vi "Meas_global.vi"() -> ()   [LabVIEW 2010]
uses:
  Controls/Board_Types.ctl
  Controls/Ch_and_Spans.ctl
  Controls/Analysis_info_cluster.ctl
  Controls/Inst_type.ctl
  Controls/Instrument_Array.ctl
  Controls/Graph_Type.ctl
  Controls/Velocity_cluster.ctl
  Controls/Correlation_cluster.ctl
  Controls/Post_Process.ctl
  Controls/Analysis_type_cluster.ctl
  Controls/Analysis_type_Enum.ctl
  Controls/Trigger_Mode.ctl
  Controls/PWA_Data.ctl
panel:
  in  "Iteration Number":i32
  in  "No of Analogue Samples":i32=128 min=0 step=1
  in  "Timescales (s)":dbl[](array[numeric]) format="%.2f"
  in  "Analogue Sampling Rate":dbl
  in  "No of Non Analogue Chs":i32
  in  "PWA Data":T1
  in  "Blocks to Skip":i32[](array[numeric])
  in  "Repeat Measurement?":bool
  in  "Duplicate channels":i32[](array[numeric])
  in  "stop":bool
  out "Flattened data type":enum16{"4.x", "Standard"}(ring)
  in  "Trigger mode":T2
  out "Time Data was Aquired":dbl format="%.2f"
  in  "No of Vari Spaced Chs":i32
  in  "Meas Setup filename":string
  in  "Error Messages":string
  in  "Extra Comments":string
  in  "Requested Sampling rate":dbl=100.0 format="%.2f"
  in  "People to Email":string[](array[string])
  in  "Actual Measurement time (min)":dbl=6.0 format="%.2f"
  in  "Averaging time (min)":dbl=6.0 format="%.2f"
  in  "Continuous time trace?":bool
  in  "Processing last block?":bool
  out "Prog's last revision date":u32
  in  "ADAM Ch Names":string[](array[string])
  in  "LDA frequency":dbl
  in  "Smoothing setups":T3(array[cluster]) {"Y axis"."Format" items=["Decimal", "Scientific", "Engineering"]; "Y axis"."Mapping" items=["Linear", "Logarithmic"]; "X axis"."Format" items=["Decimal", "Scientific", "Engineering"]; "X axis"."Mapping" items=["Linear", "Logarithmic"]}
  in  "Remote control":bool
  out "Analysis type array":T4[](array[typedef])
  out "Current Block No":i32
  in  "New Setup String":string
  in  "Analogue data":enum16{"No Analogue data", "Take Analogue data"}(ring)
  in  "Pre Setup String":string
  in  "interval scanning":bool
  in  "Post Process":T7
  in  "Transit time":bool
  in  "Arrival spacing":bool
  in  "Actual Sampling rate (Hz)":dbl=1000.0 format="%.2f"
  out "Auto-Corr control":i32[](array[numeric])
  out "Spectra control":i32[](array[numeric])
  in  "BSA data rate string":string
  in  "Cross wire + or -ve":T8(ring)
  in  "output polarity":u16(ring)=1 items=["do not change", "positive", "negative"]
  out "Correlation Cluster Array":T9[](array[typedef]) {"u^2w^2" format="%.2f"; "u^3w" format="%.2f"; "uw^3" format="%.2f"; "uw/u'w'" format="%.2f"; "uw^2" format="%.2f"; "u^2w" format="%.2f"; "uw" format="%.2f"}
  out "Velocity Cluster Array":T10[](array[typedef]) {"u^4" format="%.2f"; "Mean % Err" format="%.2f"; "u^4/(u^2)^2 -3" format="%.2f"; "u^3/(u^2)^(1.5)" format="%.2f"; "u^2" format="%.2f"; "% u'/U" format="%.2f"; "U" format="%.2f"}
  in  "LDA data":enum16{"No LDA data", "Take LDA data"}(ring)
  in  "Comments":string
  in  "Over/Under string":string
  in  "Second Graph":T12={"Plot 1"=1, "Plot 2"=3, "Save graph"=0, "Plot Type"=enum."Voltage trace"} {"Save graph" items=["Do not save plot", "Save plot"]; "Plot 2" items=["Nothing", "Velocity1", "Arr time1", "Velocity2", "Arr time2"]; "Plot 1" items=["Nothing", "Velocity1", "Arr time1", "Velocity2", "Arr time2"]}
  in  "First Graph":T12={"Plot 1"=1, "Plot 2"=3, "Save graph"=0, "Plot Type"=enum."Voltage trace"} {"Save graph" items=["Do not save plot", "Save plot"]; "Plot 2" items=["Nothing", "Velocity1", "Arr time1", "Velocity2", "Arr time2"]; "Plot 1" items=["Nothing", "Velocity1", "Arr time1", "Velocity2", "Arr time2"]}
  in  "hist extremes":dbl[][](array[numeric]) format="%.2f"
  out "Histogram control":i32[](array[numeric])
  in  "Bins":i32
  in  "Synchronise with LDA":bool
  in  "No of LDA data channels":i32
  in  "Data Validity":dbl=3.0 min=1.0 max=10.0 format="%.2f"
  out "Diagnostic info":string[][](table)
  in  "correlate":i32[][](array[numeric]) min=0 max=8
  in  "dimensions":enum16{"1D", "2D"}(ring)=enum."2D"
  in  "Raw data file":path
  in  "Analysis Info cluster":T13[](array[typedef])=[{"Colour"=0, "Inst type"=enum."Pitot-static tube", "Inst name"="Manometer voltage", "Symbol"="U", "Code name"="", "Extra Info"="U", "Inst Array"=enum."PWA", "Index"=0, "Voltage Index"=0, "Extra Titles"=[], "Extra Values"=[]}, {"Colour"=0, "Inst type"=enum."Pitot-static tube", "Inst name"="Manometer voltage", "Symbol"="U", "Code name"="", "Extra Info"="U", "Inst Array"=enum."PWA", "Index"=0, "Voltage Index"=0, "Extra Titles"=[], "Extra Values"=[]}, {"Colour"=0, "Inst type"=enum."Pitot-static tube", "Inst name"="Manometer voltage", "Symbol"="U", "Code name"="", "Extra Info"="U", "Inst Array"=enum."PWA", "Index"=0, "Voltage Index"=0, "Extra Titles"=[], "Extra Values"=[]}, {"Colour"=0, "Inst type"=enum."Pitot-static tube", "Inst name"="Manometer voltage", "Symbol"="U", "Code name"="", "Extra Info"="U", "Inst Array"=enum."PWA", "Index"=0, "Voltage Index"=0, "Extra Titles"=[], "Extra Values"=[]}]
  out "Ch & spans + mod limits":T15[](array[typedef]) {"low limit (-10V)" format="%.3f"; "high limit (10V)" format="%.3f"}
  out "Vel stat display":string[][](table)
  in  "Position":T16(array[cluster]) {"Z" format="%.1f"; "Y" format="%.1f"; "X" format="%.1f"}
  in  "Insts for plotting":u16[][](array[ring]) items=["Nothing", "Ref Prop 1", "XW1 1", "XW2 1"]
  in  "Requested No of blocks":i32
  in  "Temp":dbl=20.0 format="%.1f"
  in  "File":T17(ring)
  in  "Results file":path
  in  "Requested No of samples":i32=128 min=0 step=1
  out "Raw data option":enum16{"Save raw data", "Raw data not saved"}(ring)
  out "Start of I16 data (bytes)":i32
  in  "Start Time of experiment":dbl format="%.2f"
  out "Ch & spans":T15[](array[typedef]) {"low limit (-10V)" format="%.3f"; "high limit (10V)" format="%.3f"}
  out "Vel stats info for files":string[](array[string])
  out "Calib file strings":string[](array[string])
  out "Calib consts":dbl[][](array[numeric]) format="%.6f"
  out "Calib type name":string[](array[string])
  out "Calib files":path[](array[path])
  out "Board type":T18=enum."NB-MIO-16H"
  out "Offset voltages":dbl[](array[numeric]) format="%.2f"
  out "Abs Press (mbar)":dbl=1005.0 format="%.2f"
  out "ch info array":dbl[][](array[numeric]) format="%.2f"
  # "LDA information"
  # "File Information"
  # "Analogue input information"
  # "General controls"
  # "Analysis output information"
  # "Analysis setup information"
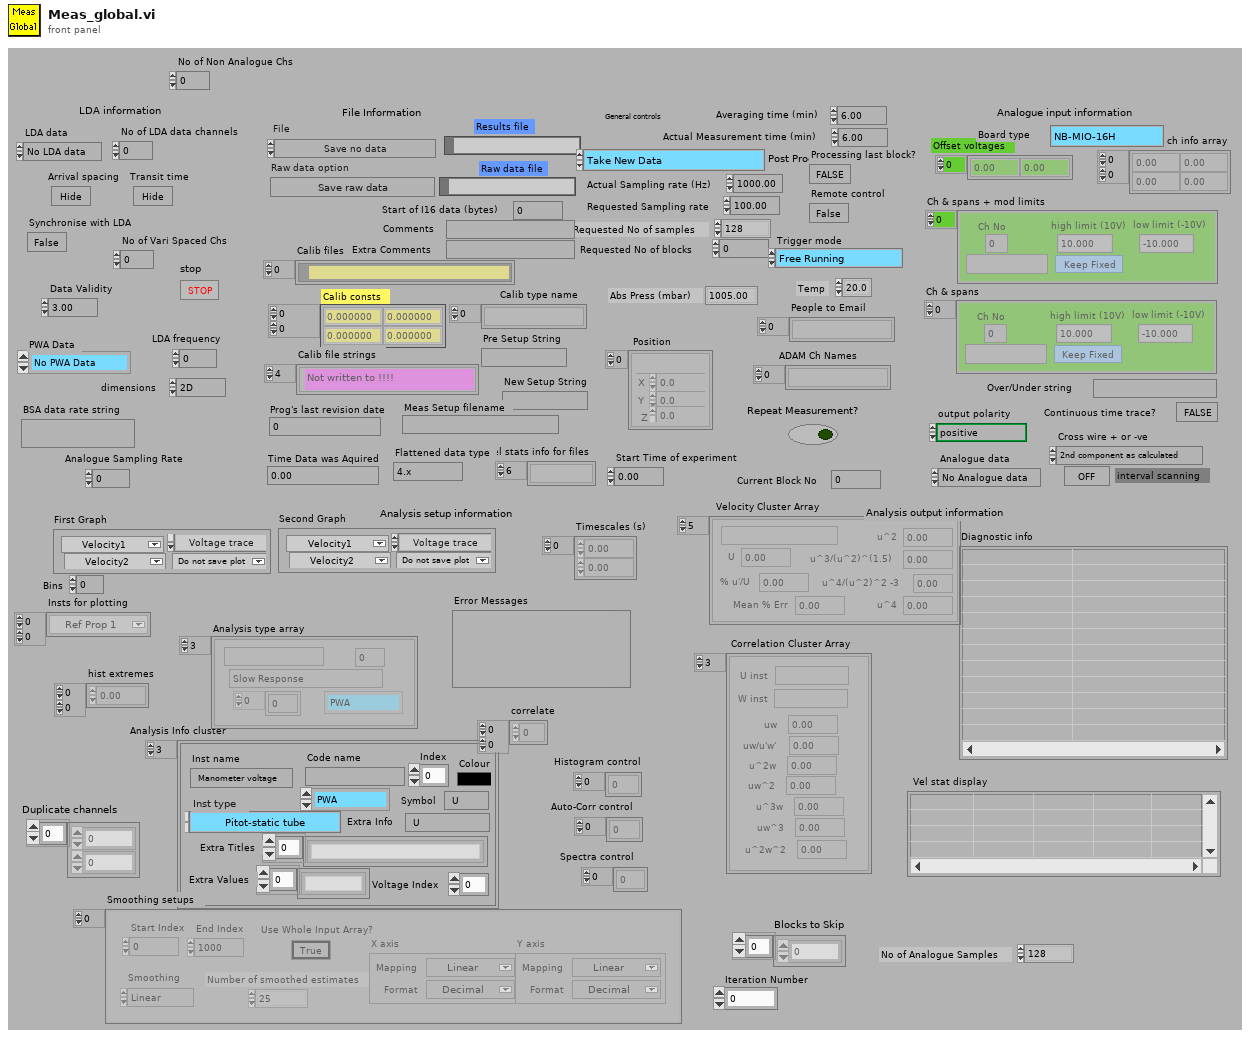
[diagram p1: front panel]
types:
  T1 = typedef "PWA_Data.ctl" = enum16{"No PWA Data", "One Ch PWA"}
  T2 = typedef "Trigger_Mode.ctl" = enum16{"Free Running", "Start on Trigger", "Trigger Every Block", "Trigger Every Sample"}
  T3 = cluster{"Start Index":i32, "End Index":i32, "Smoothing":enum16{"Linear", "Logarithmic"}, "Number of smoothed estimates":i32, "X axis":cluster{"Mapping":u16, "Format":u16}, "Y axis":cluster{"Mapping":u16, "Format":u16}, "Use Whole Input Array?":bool}[]
  T4 = typedef "Analysis_type_cluster.ctl" = cluster{"Analysis type":T5, "Indicies":i32[], "Name":string, "Inst Array":T6, "Info index":i32}
  T5 = typedef "Analysis_type_Enum.ctl" = enum16{"Slow Response", "Fast Response", "Weighted Fast Response", "Fast FID", "Weighted Fast FID", "Cross Wire", "Weighted Cross Wire", "Weighted LDA"}
  T6 = typedef "Instrument_Array.ctl" = enum16{"PWA", "LDA", "Analogue"}
  T7 = typedef "Post_Process.ctl" = enum16{"Take New Data", "Post Process Raw Data File"}
  T8 = enum16{"2nd component as calculated", "2nd component multipled by -1"}
  T9 = typedef "Correlation_cluster.ctl" = cluster{"U inst":string, "W inst":string, "uw":dbl, "uw/u'w'":dbl, "u^2w":dbl, "uw^2":dbl, "uw^3":dbl, "u^3w":dbl, "u^2w^2":dbl}
  T10 = typedef "Velocity_cluster.ctl" = cluster{"Name":string, "U":dbl, "u^2":dbl, "u^3/(u^2)^(1.5)":dbl, "u^4/(u^2)^2 -3":dbl, "% u'/U":dbl, "Mean % Err":dbl, "u^4":dbl}
  T11 = typedef "Graph_Type.ctl" = enum16{"Show no graph", "Voltage trace", "Velocity trace", "Vel histogram", "Spectrum", "f.E(f) v Log f", "Auto-Corr"}
  T12 = cluster{"Plot 1":u16, "Plot 2":u16, "Save graph":u16, "Plot Type":T11}
  T13 = typedef "Analysis_info_cluster.ctl" = cluster{"Colour":u32, "Inst type":T14, "Inst name":string, "Symbol":string, "Code name":string, "Extra Info":string, "Inst Array":T6, "Index":i32, "Voltage Index":i32, "Extra Titles":string[], "Extra Values":string[]}
  T14 = typedef "Inst_type.ctl" = enum16{"Propeller anemometer", "Raw voltage", "Pressure Transducer", "Pitot-static tube", "Preston tube", "Hot wire", "Cross wire 1", "Cross wire 2", "Generic Linear", "Generic Polynomial", "Generic BackPoly", "Fast FID", "Thermocouple", "Cold wire", "Pulsed Wire", "LDA Vel", "LDA Tran time", "LDA Arr time"}
  T15 = typedef "Ch_and_Spans.ctl" = cluster{"high limit (10V)":sgl, "low limit (-10V)":sgl, "Ch No":i16, "Var name":string, "Use Latest Calib":bool}
  T16 = cluster{"Name":string, "X":dbl, "Y":dbl, "Z":dbl}[]
  T17 = enum16{"Save no data", "Save data in new files", "Save data in existing files"}
  T18 = typedef "Board_Types.ctl" = enum16{"Simulate", "NB-MIO-16H", "PCI-MIO-16E", "6000E Series", "USB-92xx", "ADC488", "Lab-NB", "NB-DIO-24", "NI-DAQmx", "Local ADAM", "Server Channels"}
diagram:
